vi "5_Waveform Parameters.vi"(0 "Test No":T1) -> (1 "Sample Rate (Samples/sec)":dbl[](array[numeric])=[nan, nan, nan, nan, nan, nan], 4 "Frequency Index":dbl[](array[numeric])=[nan, nan, nan, nan, nan, nan], 5 "Frequency (Hz)":dbl[](array[numeric])=[nan, nan, nan, nan, nan, nan], 6 "Stim Amplitude (mA)":dbl[](array[numeric])=[nan, nan, nan, nan, nan, nan], 7 "CBC Holdoff (µs)":dbl[](array[numeric])=[nan, nan, nan, nan, nan, nan], 10 "Samples":dbl[](array[numeric])=[nan, nan, nan, nan, nan, nan], 11 "Digitizer Range":dbl[](array[numeric])=[nan, nan, nan, nan, nan, nan], 12 "Stim Pulse Width (µs)":dbl[](array[numeric])=[nan, nan, nan, nan, nan, nan], 13 "CBC width (µs)":dbl[](array[numeric])=[nan, nan, nan, nan, nan, nan], 14 "Interphase Delay (µs)":dbl[](array[numeric])=[nan, nan, nan, nan, nan, nan], 15 "Active Recovery Amp (mA)":dbl[](array[numeric])=[nan, nan, nan, nan, nan, nan], 16 "Average Size":dbl[](array[numeric])=[nan, nan, nan, nan, nan, nan], 17 "Recovery Ratio Krec":dbl[](array[numeric])=[nan, nan, nan, nan, nan, nan], 18 "Active/Passive Recovery PW (µs)":dbl[](array[numeric])=[nan, nan, nan, nan, nan, nan], 19 "Active/Passive Holdoff  (µs)":dbl[](array[numeric])=[nan, nan, nan, nan, nan, nan])   [LabVIEW 2010]
uses:
  5_Waveform Parameters Test No.ctl
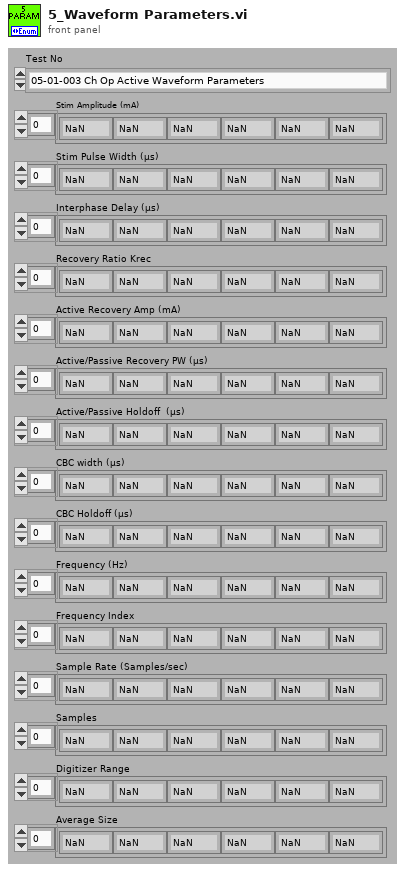
[diagram p1: front panel]
types:
  T1 = typedef "5_Waveform Parameters Test No.ctl" = enum16{"05-01-003 Ch Op Active Waveform Parameters", "05-01-004 Enclosure Op Active Waveform Parameters"}
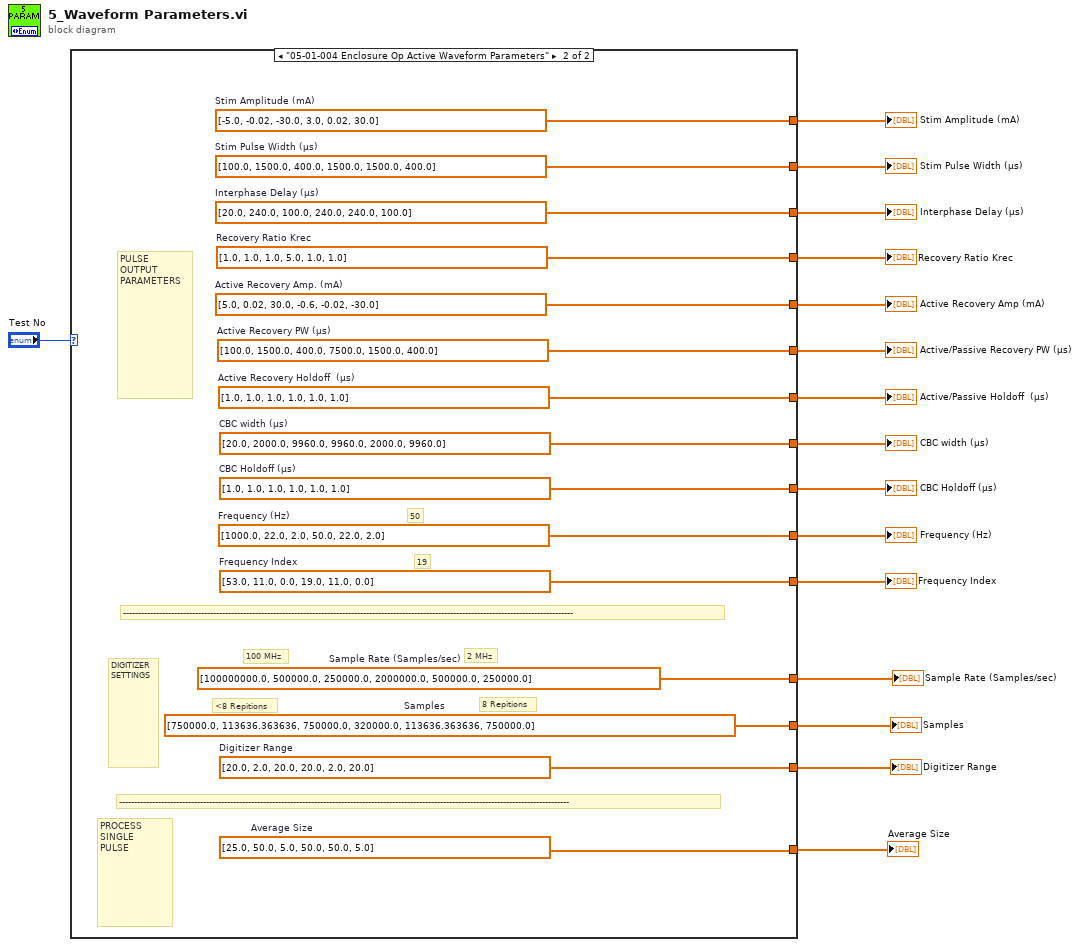
[diagram p0: block diagram]
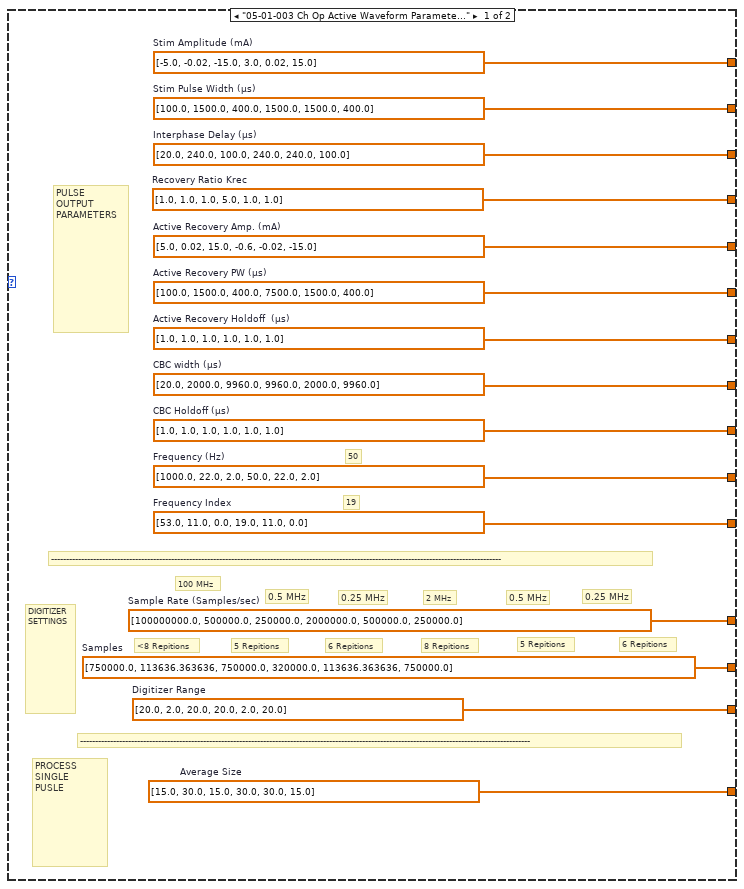
[diagram p2: hidden frame]
diagram:
  n1 = case shown="\"05-01-004 Enclosure Op Active Waveform Parameters\"" "Test No" {
    tunnel: [w31 w46] -> w16
    tunnel: [w30 w45] -> w15
    tunnel: [w29 w44] -> w14
    tunnel: [w28 w43] -> w13
    tunnel: [w27 w42] -> w12
    tunnel: [w26 w41] -> w11
    tunnel: [w25 w40] -> w10
    tunnel: [w24 w39] -> w9
    tunnel: [w23 w38] -> w8
    tunnel: [w22 w37] -> w7
    tunnel: [w21 w36] -> w5
    tunnel: [w20 w35] -> w4
    tunnel: [w19 w34] -> w3
    tunnel: [w18 w33] -> w2
    tunnel: [w17 w32] -> w1
    frame "05-01-003 Ch Op Active Waveform Parameters" {
      w17 = dbl[] [1.0, 1.0, 1.0, 5.0, 1.0, 1.0]  # Recovery Ratio Krec
      w18 = dbl[] [15.0, 30.0, 15.0, 30.0, 30.0, 15.0]  # Average Size
      w19 = dbl[] [20.0, 2.0, 20.0, 20.0, 2.0, 20.0]  # Digitizer Range
      w20 = dbl[] [750000.0, 113636.363636, 750000.0, 320000.0, 113636.363636, 750000.0]  # Samples
      w21 = dbl[] [5.0, 0.02, 15.0, -0.6, -0.02, -15.0]  # Active Recovery Amp. (mA)
      w22 = dbl[] [100000000.0, 500000.0, 250000.0, 2000000.0, 500000.0, 250000.0]  # Sample Rate (Samples/sec)
      w23 = dbl[] [53.0, 11.0, 0.0, 19.0, 11.0, 0.0]  # Frequency Index
      w24 = dbl[] [1000.0, 22.0, 2.0, 50.0, 22.0, 2.0]  # Frequency (Hz)
      w25 = dbl[] [1.0, 1.0, 1.0, 1.0, 1.0, 1.0]  # CBC Holdoff (µs)
      w26 = dbl[] [20.0, 2000.0, 9960.0, 9960.0, 2000.0, 9960.0]  # CBC width (µs)
      w27 = dbl[] [1.0, 1.0, 1.0, 1.0, 1.0, 1.0]  # Active Recovery Holdoff  (µs)
      w28 = dbl[] [100.0, 1500.0, 400.0, 7500.0, 1500.0, 400.0]  # Active Recovery PW (µs)
      w29 = dbl[] [20.0, 240.0, 100.0, 240.0, 240.0, 100.0]  # Interphase Delay (µs)
      w30 = dbl[] [100.0, 1500.0, 400.0, 1500.0, 1500.0, 400.0]  # Stim Pulse Width (µs)
      w31 = dbl[] [-5.0, -0.02, -15.0, 3.0, 0.02, 15.0]  # Stim Amplitude (mA)
      # "50"
      # "19"
      # "------------------------------------------------------------------------------------------------------------------------------------------------------"
      # "6 Repitions"
      # "0.25 MHz"
      # "2 MHz"
      # "8 Repitions"
      # "5 Repitions"
      # "6 Repitions"
      # "0.25 MHz"
      # "5 Repitions"
      # "<8 Repitions"
      # "0.5 MHz"
      # "100 MHz"
      # "0.5 MHz"
      # "------------------------------------------------------------------------------------------------------------------------------------------------------"
      # "PROCESS\nSINGLE\nPUSLE"
      # "DIGITIZER\nSETTINGS"
      # "PULSE\nOUTPUT\nPARAMETERS"
    }
    frame "05-01-004 Enclosure Op Active Waveform Parameters" {
      w32 = dbl[] [1.0, 1.0, 1.0, 5.0, 1.0, 1.0]  # Recovery Ratio Krec
      w33 = dbl[] [25.0, 50.0, 5.0, 50.0, 50.0, 5.0]  # Average Size
      w34 = dbl[] [20.0, 2.0, 20.0, 20.0, 2.0, 20.0]  # Digitizer Range
      w35 = dbl[] [750000.0, 113636.363636, 750000.0, 320000.0, 113636.363636, 750000.0]  # Samples
      w36 = dbl[] [5.0, 0.02, 30.0, -0.6, -0.02, -30.0]  # Active Recovery Amp. (mA)
      w37 = dbl[] [100000000.0, 500000.0, 250000.0, 2000000.0, 500000.0, 250000.0]  # Sample Rate (Samples/sec)
      w38 = dbl[] [53.0, 11.0, 0.0, 19.0, 11.0, 0.0]  # Frequency Index
      w39 = dbl[] [1000.0, 22.0, 2.0, 50.0, 22.0, 2.0]  # Frequency (Hz)
      w40 = dbl[] [1.0, 1.0, 1.0, 1.0, 1.0, 1.0]  # CBC Holdoff (µs)
      w41 = dbl[] [20.0, 2000.0, 9960.0, 9960.0, 2000.0, 9960.0]  # CBC width (µs)
      w42 = dbl[] [1.0, 1.0, 1.0, 1.0, 1.0, 1.0]  # Active Recovery Holdoff  (µs)
      w43 = dbl[] [100.0, 1500.0, 400.0, 7500.0, 1500.0, 400.0]  # Active Recovery PW (µs)
      w44 = dbl[] [20.0, 240.0, 100.0, 240.0, 240.0, 100.0]  # Interphase Delay (µs)
      w45 = dbl[] [100.0, 1500.0, 400.0, 1500.0, 1500.0, 400.0]  # Stim Pulse Width (µs)
      w46 = dbl[] [-5.0, -0.02, -30.0, 3.0, 0.02, 30.0]  # Stim Amplitude (mA)
      # "19"
      # "50"
      # "8 Repitions"
      # "<8 Repitions"
      # "2 MHz"
      # "100 MHz"
      # "------------------------------------------------------------------------------------------------------------------------------------------------------"
      # "------------------------------------------------------------------------------------------------------------------------------------------------------"
      # "DIGITIZER\nSETTINGS"
      # "PULSE\nOUTPUT\nPARAMETERS"
      # "PROCESS\nSINGLE\nPULSE"
    }
  }
  "Stim Amplitude (mA)" <- w16
  "Stim Pulse Width (µs)" <- w15
  "Interphase Delay (µs)" <- w14
  "Active/Passive Recovery PW (µs)" <- w13
  "Active/Passive Holdoff  (µs)" <- w12
  "CBC width (µs)" <- w11
  "CBC Holdoff (µs)" <- w10
  "Frequency (Hz)" <- w9
  "Frequency Index" <- w8
  "Sample Rate (Samples/sec)" <- w7
  "Active Recovery Amp (mA)" <- w5
  "Samples" <- w4
  "Digitizer Range" <- w3
  "Average Size" <- w2
  "Recovery Ratio Krec" <- w1
